vi "Release Timeout Notifier.vi"(8 "error in (no error)":errorcluster, 11 "State Actor in":refnum<class "State Actor.lvclass">) -> (0 "error out":errorcluster, 3 "State Actor out":refnum<class "State Actor.lvclass">)   [LabVIEW 2024, in "State Actor.lvlib" / "State Actor.lvclass"]
uses:
  State Actor.lvclass
  State Actor.lvclass/State Actor.ctl
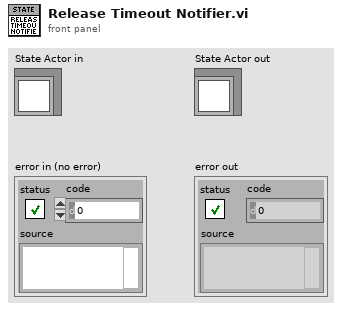
[diagram p1: front panel]
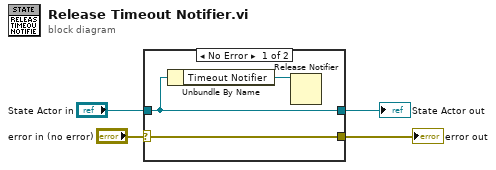
[diagram p0: block diagram]
diagram:
  n1 = case shown="No Error" "error in (no error)" {
    selector: "error in (no error)" -> [w5 w9]
    tunnel: [w5 w9] -> w3
    tunnel: [w7 w8] -> w1
    tunnel: "State Actor in" -> [w7 w8]
    frame No Error {
      n2 = Unbundle By Name(w7) -> ("Timeout Notifier"=w6:refnum<notifier>)
      n3 = Release Notifier(notifier=w6) -> ()  [unwired: 2 in, 3 out]
    }
    frame Error {
    }
  }
  "error out" <- w3
  "State Actor out" <- w1
